vi "ex8-7_new.vi"   [LabVIEW 2013]
uses:
  <vilib>/NXT/Block Support/NXT_MessageMailbox.ctl
  <vilib>/NXT/NXT Controls/ConnectionType.ctl
  <vilib>/NXT/Dual Mode Library/BT/BlueTooth_Write_String_c2.vi
types:
  T1 = typedef "ConnectionType.ctl" = enum16{"Bluetooth", "USB", "WiFi"}
  T2 = typedef "NXT_MessageMailbox.ctl" = u8
  T3 = typedef "LVHSConnector.ctl" = refnum<class "BrickReference.lvclass">
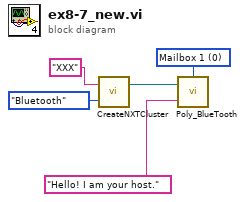
[diagram p0: block diagram]
diagram:
  w5 = T2 0 items=["Mailbox 1", "Mailbox 2", "Mailbox 3", "Mailbox 4", "Mailbox 5", "Mailbox 6", "Mailbox 7", "Mailbox 8", "Mailbox 9", "Mailbox 10"] ("Mailbox")
  n1 = call <vilib>:"CreateNXTCluster.vi"("Connection Type"=ConnectionType."Bluetooth", "NXT/EV3 name"="XXX") -> ("NXT/EV3"=w3:T3)  [unwired: 2 in]
  n2 = call-poly <vilib>:"Poly_BlueTooth.vi"("Message"="Hello! I am your host.", "NXT/EV3"=w3, "Mailbox"=w5) -> ()  [unwired: 1 in, 1 out]
